vi "Robot Main.vi"() -> ()   [LabVIEW 2017]
doc: "Robot Main serves as the primary scheduler for your command and control robotics program. It should not be necessary to modify this VI. Instead, you should add your code to the VIs called from Robot Main - Teleop, Autonomous, and SubSystems."
uses:
  <vilib>/Rock Robotics/WPI/Camera/WPI_CameraImageSize.ctl
  <vilib>/Rock Robotics/WPI/DriverStation/WPI_DriverStationPositionInfo.ctl
  <vilib>/Rock Robotics/SystemInterfaces/NetworkCommunication/NetComm_UsageReport_ResourceType.ctl
  Framework/Robot Global Data.vi
panel:
  in  "Auto Type":bool=TRUE
  in  "Auto Raise Arm Time (ms)":dbl=1000.0
  in  "Auto Lower Cube Time (ms)":dbl=1000.0
  in  "Auto Release CubeTime (ms)":dbl=1000.0
  in  "Switch Position":string="R" caption="L = Left\nR = Right"
  in  "Robot Position":T1=enum."2" caption="1 = Left\n2 = Middle\n3 = Right"
  in  "Hook Down Time (ms)":dbl=200.0
  in  "Hook Up Time (ms)":dbl=200.0
  in  "Backward Time (ms)":dbl=20.0
  in  "Forward Time (ms)":dbl=20.0
  in  "Hook Arm Down Time (ms)":dbl=200.0
  in  "Hook Arm Up Time (ms)":dbl=200.0
  in  "Right Turn Time (ms)":dbl=20.0
  in  "Left Turn Time (ms)":dbl=20.0
  in  "Rate reduction":dbl=0.9
  in  "Min Output(0 to 1)":dbl=0.8
  in  "Select Mode":T2(ring)=enum."Square with Rate"
  in  "n^x(Unbounded)":dbl=3.0 format="%#_13g"
  in  "Image Size":T3=enum."320x240"
  in  "Enable Vision":bool=TRUE
  in  "Finish":bool
  # "Auto Settings"
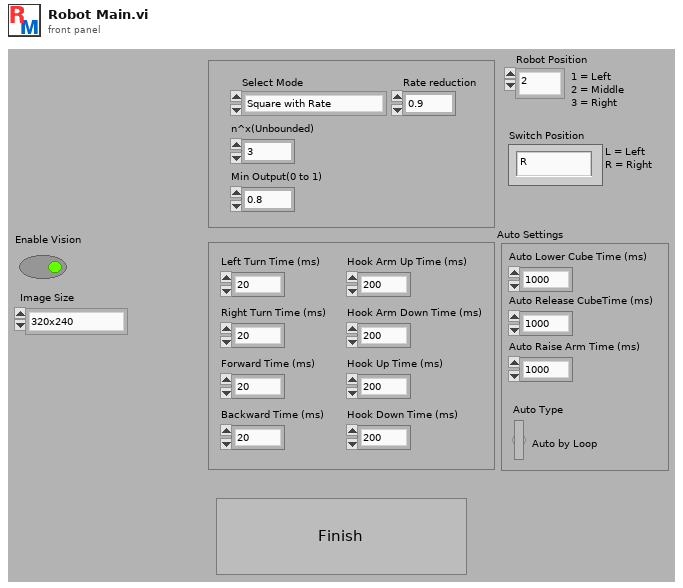
[diagram p1: front panel]
types:
  T1 = typedef "WPI_DriverStationPositionInfo.ctl" = enum16{"1", "2", "3"}
  T2 = enum16{"Normal", "Square", "Square with Rate", "Square Root", "Linear", "Exponential"}
  T3 = typedef "WPI_CameraImageSize.ctl" = enum16{"640x480", "320x240", "160x120", "Custom"}
  T4 = typedef "NetComm_UsageReport_ResourceType.ctl" = enum8{"Controller", "Module", "Language", "CANPlugin", "Accelerometer", "ADXL345", "AnalogChannel", "AnalogTrigger", "AnalogTriggerOutput", "CANJaguar", "Compressor", "Counter", "Dashboard", "DigitalInput", "DigitalOutput", "DriverStationCIO", "DriverStationEIO", "DriverStationLCD", "Encoder", "GearTooth", "Gyro", "I2C", "Framework", "Jaguar", "Joystick", "Kinect", "KinectStick", "PIDController", "Preferences", "PWM", "Relay", "RobotDrive", "SerialPort", "Servo", "Solenoid", "SPI", "Task", "Ultrasonic", "Victor", "Button", "Command", "AxisCamera", "PCVideoServer", "SmartDashboard", "Talon", "HiTechnicColorSensor", "HiTechnicAccel", "HiTechnicCompass", "SRF08", "AnalogOutput", "Victor SP", "Talon SRX", "CAN Talon SRX", "ADXL362 Accel", "ADXRS450 Gyro", "Rev SPARK", "Mindsensors SD540", "Digital Filter", "ADIS16448", "PDP", "PCM", "PigeonIMU", "Nidec Brushless", "CTRE CANifier", "CTRE Future 0", "CTRE Future 1", "CTRE Future 2", "CTRE Future 3", "CTRE Future 4", "CTRE Future 5", "CTRE Future 6"}
  T5 = typedef "WPI_DriverStationMatch Info.ctl" = cluster{"Autonomous Elapsed Seconds":dbl, "TeleOp Elapsed Seconds":dbl, "Disabled Elapsed Seconds":dbl, "Visited Autonomous":bool, "Visited TeleOp":bool, "Visited Disabled":bool, "Autonomous Settings":cluster{"Autonomous Style":enum16{"Iterative", "Independent"}, "VI Refnum":refnum<vi>}}
  T6 = typedef "WPI_DriverStationDerivedRobotMode.ctl" = enum16{"Init", "Execute", "Stop"}
  T7 = typedef "WPI_DriverStationRobotMode2.ctl" = enum16{"Autonomous Disabled", "Autonomous Enabled", "Teleop Disabled", "Teleop Enabled", "Disconnected", "Finish", "Test Disabled", "Test Enabled", "Emergency Stopped"}
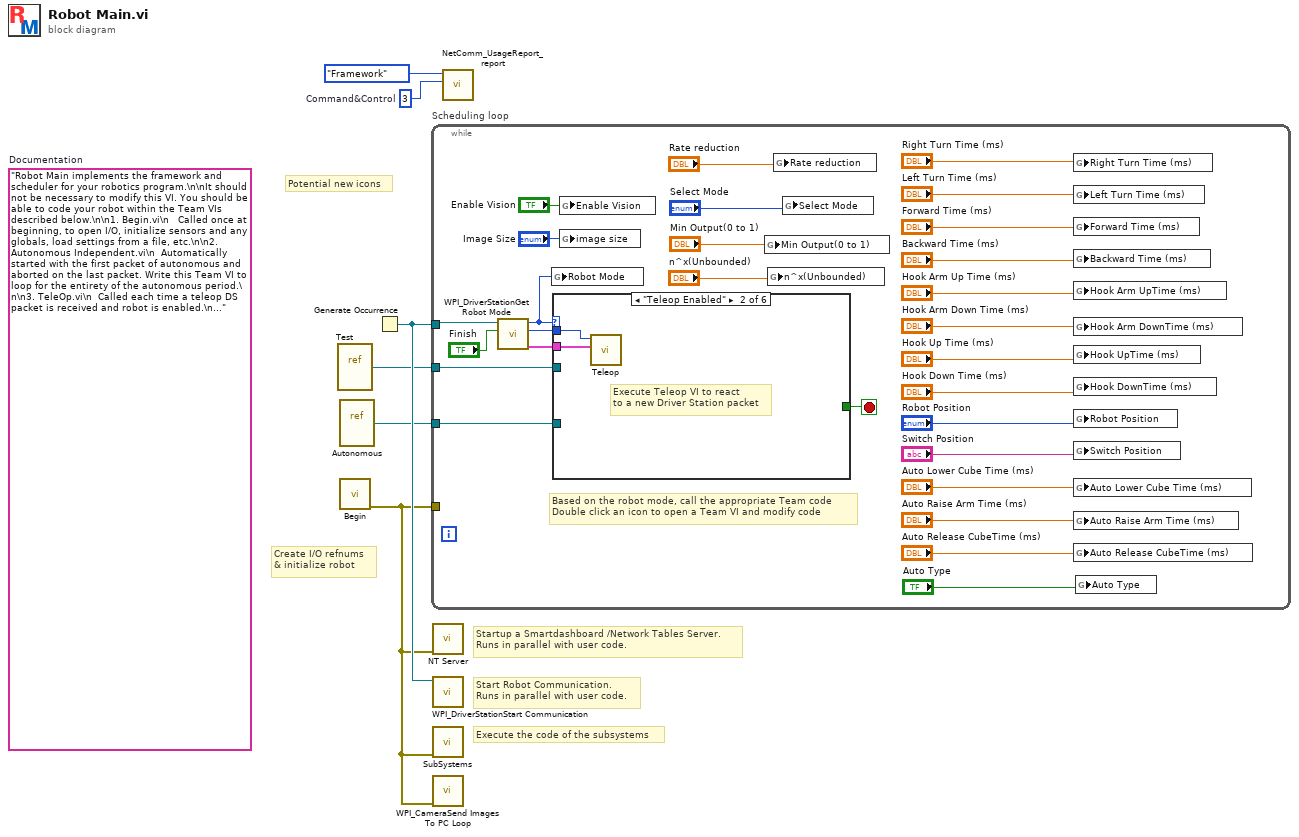
[diagram p0: block diagram]
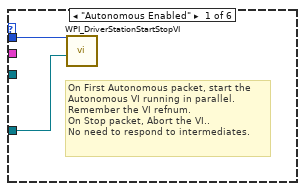
[diagram p2: hidden frame]
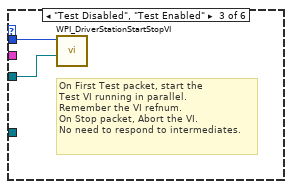
[diagram p3: hidden frame]
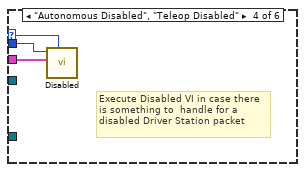
[diagram p4: hidden frame]
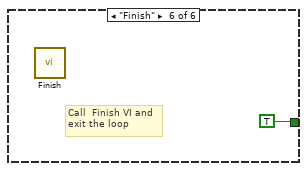
[diagram p6: hidden frame]
diagram:
  w2 = u8 3  # Command&Control
  (unwired) "Robot Main implements the framework and scheduler for your robotics program.\n\nIt should not be necessary to modify this VI. You should be able to code your robot within the Team VIs described below.\n\n1. Begin.vi\n   Called once at beginning, to open I/O, initialize sensors and any globals, load settings from a file, etc.\n\n2. Autonomous Independent.vi\n  Automatically started with the first packet of autonomous and aborted on the last packet. Write this Team VI to loop for the entirety of the autonomous period.\n\n3. TeleOp.vi\n  Called each time a teleop DS packet is received and robot is enabled.\n\n4. Disabled.vi\n  Called each time a packet is received and the robot is disabled.\n\n5. Test.vi\n  Called Automatically started with the first test packet and aborted on the last. Modify this VI to carry out robot and sensor validation tests.\n\n6. Vision.vi\n  A parallel loop that acquires and processes camera images.\n\n7. PeriodicTasks.vi\n  Parallel loops running at user-defined rates.\n\n8. Finish.vi\n  Called before exiting, so you can save data, clean up I/O, etc.\n"  # Documentation
  # "Potential new icons"
  # "Startup a Smartdashboard /Network Tables Server.\nRuns in parallel with user code."
  # "Execute the code of the subsystems"
  # "Create I/O refnums\n& initialize robot"
  # "Start Robot Communication.\nRuns in parallel with user code."
  n1 = vi-ref "Test.vi"() -> (w4:refnum<vi>)
  n2 = vi-ref "Autonomous.vi"() -> (w5:refnum<vi>)
  n3 = call "Begin.vi"() -> ("error out"=w1:errorcluster)  [unwired: 2 in, 9 out]
  n4 = Generate Occurrence() -> (w6:refnum<k4>)
  n5 = while "Scheduling loop" {
    tunnel: w6 -> [w33]
    tunnel: w1 -> [_]
    tunnel: w5 -> [w28]
    tunnel: w4 -> [w26]
    stop <- w30 stop-if-true
    # "Based on the robot mode, call the appropriate Team code\nDouble click an icon to open a Team VI and modify code"
    n6 = call <vilib>:"WPI_DriverStationGet Robot Mode.vi"("Finish"="Finish", "DS Occurrence"=w33) -> ("Match Info out"=w31:T5, "Call Context"=w34:T6, "Robot Mode"=w25:T7)  [unwired: 7 out]
    n7 = global write "Robot Global Data.vi" "Robot Mode"(w25) -> ()
    n8 = case shown="\"Teleop Enabled\"" w25 {
      selector: w25 -> [_ _ _ w41 _ _]
      tunnel: w34 -> [w36 w38 w40 w43 _ _]
      tunnel: w31 -> [_ w37 _ w42 _ _]
      tunnel: [_ _ _ _ _ TRUE] -> w30
      tunnel: w28 -> [w35 _ _ _ _ _]
      tunnel: w26 -> [_ _ w39 _ _ _]
      frame "Autonomous Enabled" {
        # "On First Autonomous packet, start the\nAutonomous VI running in parallel.\nRemember the VI refnum.\nOn Stop packet, Abort the VI..\nNo need to respond to intermediates."
        n9 = call <vilib>:"WPI_DriverStationStartStopVI.vi"("VI in"=w35, "Call Context"=w36) -> ()  [unwired: 10 in]
      }
      frame "Teleop Enabled" {
        # "Execute Teleop VI to react\nto a new Driver Station packet"
        n10 = call "Teleop.vi"("Match Info"=w37, "Call Context"=w38) -> ()  [unwired: 1 in, 9 out]
      }
      frame "Test Disabled", "Test Enabled" {
        # "On First Test packet, start the\nTest VI running in parallel.\nRemember the VI refnum.\nOn Stop packet, Abort the VI.\nNo need to respond to intermediates."
        n11 = call <vilib>:"WPI_DriverStationStartStopVI.vi"("VI in"=w39, "Call Context"=w40) -> ()  [unwired: 10 in]
      }
      frame "Autonomous Disabled", "Teleop Disabled" {
        # "Execute Disabled VI in case there\nis something to  handle for a\ndisabled Driver Station packet"
        n12 = call "Disabled.vi"("Robot Mode"=w41, "Match Info"=w42, "Call Context"=w43) -> ()  [unwired: 1 in, 8 out]
      }
      frame "Disconnected", Default {
        # "Driver Station packet didn't arrive.\nPossibly useful for diagnostics"
      }
      frame "Finish" {
        # "Call  Finish VI and\nexit the loop"
        n13 = call "Finish.vi"() -> ()  [unwired: 1 in, 7 out]
      }
    }
    n14 = global write "Robot Global Data.vi" "Enable Vision"("Enable Vision") -> ()
    n15 = global write "Robot Global Data.vi" "image size"("Image Size") -> ()
    n16 = global write "Robot Global Data.vi" "Min Output(0 to 1)"("Min Output(0 to 1)") -> ()
    n17 = global write "Robot Global Data.vi" "n^x(Unbounded)"("n^x(Unbounded)") -> ()
    n18 = global write "Robot Global Data.vi" "Rate reduction"("Rate reduction") -> ()
    n19 = global write "Robot Global Data.vi" "Select Mode"("Select Mode") -> ()
    n20 = global write "Robot Global Data.vi" "Right Turn Time (ms)"("Right Turn Time (ms)") -> ()
    n21 = global write "Robot Global Data.vi" "Left Turn Time (ms)"("Left Turn Time (ms)") -> ()
    n22 = global write "Robot Global Data.vi" "Forward Time (ms)"("Forward Time (ms)") -> ()
    n23 = global write "Robot Global Data.vi" "Backward Time (ms)"("Backward Time (ms)") -> ()
    n24 = global write "Robot Global Data.vi" "Hook Arm UpTime (ms)"("Hook Arm Up Time (ms)") -> ()
    n25 = global write "Robot Global Data.vi" "Hook Arm DownTime (ms)"("Hook Arm Down Time (ms)") -> ()
    n26 = global write "Robot Global Data.vi" "Hook UpTime (ms)"("Hook Up Time (ms)") -> ()
    n27 = global write "Robot Global Data.vi" "Hook DownTime (ms)"("Hook Down Time (ms)") -> ()
    n28 = global write "Robot Global Data.vi" "Robot Position"("Robot Position") -> ()
    n29 = global write "Robot Global Data.vi" "Switch Position"("Switch Position") -> ()
    n30 = global write "Robot Global Data.vi" "Auto Lower Cube Time (ms)"("Auto Lower Cube Time (ms)") -> ()
    n31 = global write "Robot Global Data.vi" "Auto Raise Arm Time (ms)"("Auto Raise Arm Time (ms)") -> ()
    n32 = global write "Robot Global Data.vi" "Auto Release CubeTime (ms)"("Auto Release CubeTime (ms)") -> ()
    n33 = global write "Robot Global Data.vi" "Auto Type"("Auto Type") -> ()
  }
  n34 = call <vilib>:"NT Server.vi"("error in (no error)"=w1) -> ()  [unwired: 11 in]
  n35 = call <vilib>:"WPI_DriverStationStart Communication.vi"("occurrence"=w6) -> ()  [unwired: 1 in, 10 out]
  n36 = call "SubSystems.vi"("error in"=w1) -> ()  [unwired: 11 in]
  n37 = call <vilib>:"WPI_CameraSend Images To PC Loop.vi"("error in (no error)"=w1) -> ()  [unwired: 11 in]
  n38 = call <vilib>:"NetComm_UsageReport_report.vi"("Instance Number"=w2, "Resource Type"=NetComm_UsageReport_ResourceType."Framework") -> ()  [unwired: 10 in]
